vi "SetHeight.vi"(10 "Height":dbl, 11 "Rectangle In":refnum<class "Rectangle.lvclass">) -> (3 "Rectangle Out":refnum<class "Rectangle.lvclass">)   [LabVIEW 2018, in "Rectangle.lvclass"]
uses:
  Rectangle.lvclass
  Rectangle.lvclass/Rectangle.ctl
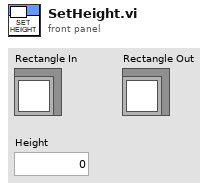
[diagram p1: front panel]
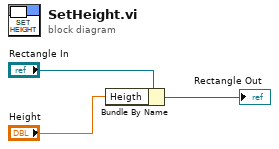
[diagram p0: block diagram]
diagram:
  n1 = Bundle By Name(cluster="Rectangle In", "Heigth"="Height") -> (→"Rectangle Out":refnum<class "Rectangle.lvclass">)
